vi "Write2VISA.vi"(8 "error in (no error)":errorcluster, 10 "Message_command In":T1, 11 "Command Queue In":T2) -> (0 "error out":errorcluster, 2 "Message_command Out":T1, 3 "Command Queue out":T2)   [LabVIEW 2020]
uses:
  Command_Queue.ctl
  Command_Message.ctl
  <vilib>/regexp/Match Regular Expression.xnode
panel:
  out "concatenated string":string
  out "Command":string
  out "VISA instruments":refnum<visa-resource-name>
  in  "VISA instruments":string[](array[string])=["gpib", "asrl", "com", "end of list"]
  # "end of list should be the last item"
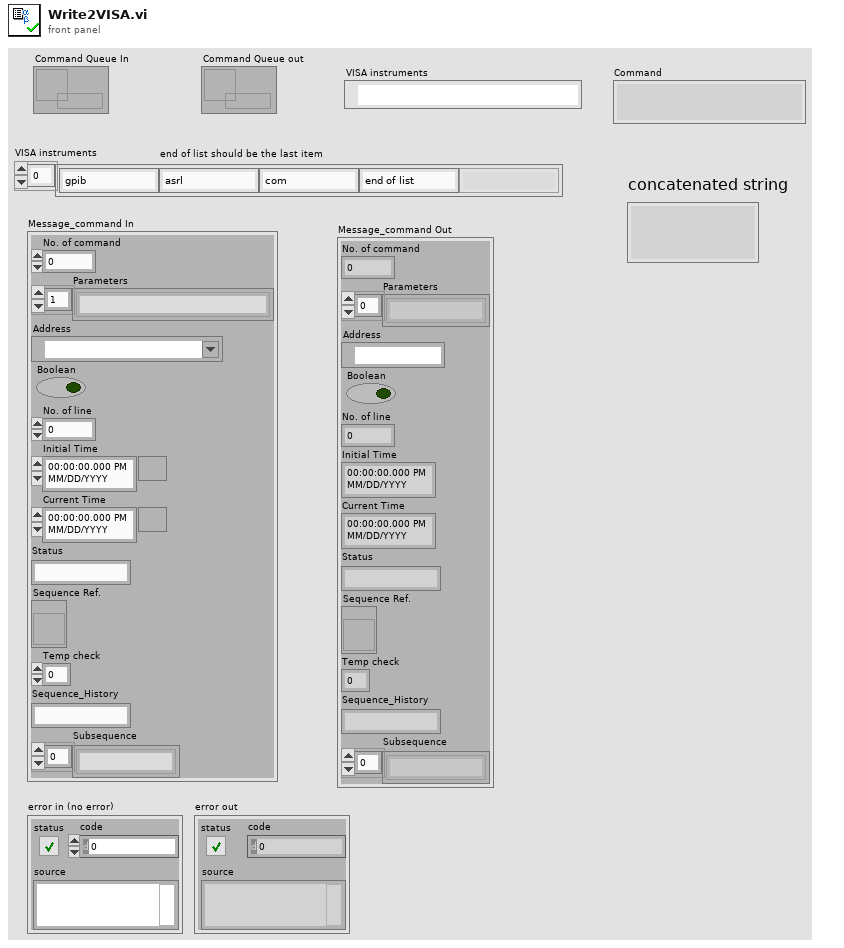
[diagram p1: front panel]
types:
  T1 = typedef "Command_Message.ctl" = cluster{"No. of command":i32, "Parameters":string[], "Address":refnum<visa-resource-name>, "Boolean":bool, "No. of line":i32, "Initial Time":timestamp, "Current Time":timestamp, "Status":string, "Sequence Ref.":refnum<vi>, "Temp check":i32, "Sequence_History":string, "Subsequence":string[]}
  T2 = typedef "Command_Queue.ctl" = refnum<queue>
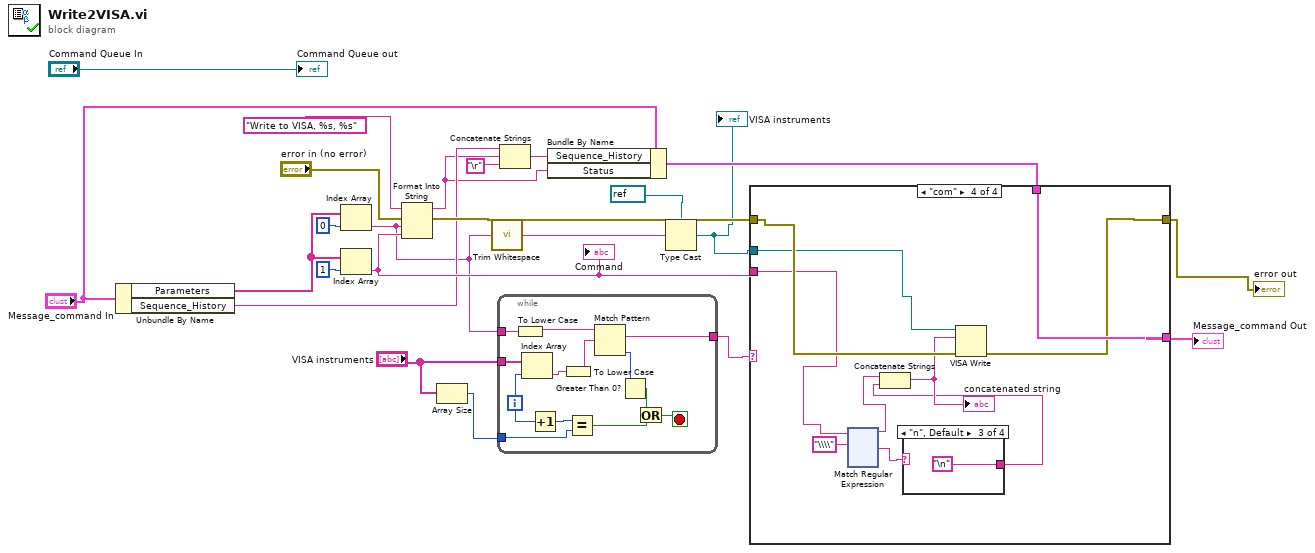
[diagram p0: block diagram]
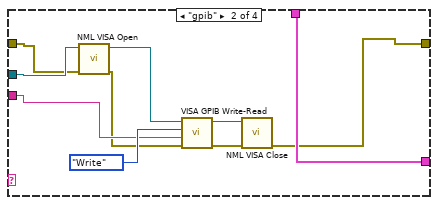
[diagram p3: hidden frame]
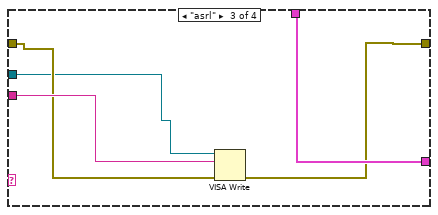
[diagram p4: hidden frame]
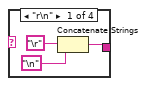
[diagram p5: hidden frame]
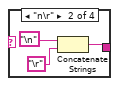
[diagram p6: hidden frame]
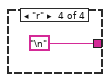
[diagram p7: hidden frame]
diagram:
  n1 = Unbundle By Name("Message_command In") -> ("Parameters"=w21:string[], "Sequence_History"=w15:string)
  n2 = Index Array(array=w21, index=0) -> (element=w5:string)
  n3 = Index Array(array=w21, index=1) -> (element=w18:string)
  "Command" <- w18
  n4 = Format Into String(format string="Write to VISA, %s, %s", error in="error in (no error)", w5, w18) -> (resulting string=w12:string, error out=w17:errorcluster)  [unwired: 1 in]
  n5 = Array Size(array="VISA instruments") -> (size(s)=w6:i32)
  n6 = call <vilib>:"Trim Whitespace.vi"("string"=w5) -> ("trimmed string"=w2:string)  [unwired: 1 in]
  n7 = while {
    tunnel: w5 -> [w36]
    tunnel: "VISA instruments" -> [w35]
    tunnel: [w30] -> w3
    tunnel: w6 -> [w25]
    i -> [w27]
    stop <- w28 stop-if-true
    n8 = To Lower Case(string=w36) -> (all lower case string=w32:string)
    n9 = Index Array(array=w35, index=w27) -> (element=w34:string)
    n10 = Increment(x=w27) -> (x+1=w26:i32)
    n11 = To Lower Case(string=w34) -> (all lower case string=w33:string)
    n12 = Equal?(x=w26, y=w25) -> (x = y?=w24:bool)
    n13 = Match Pattern(string=w32, regular expression=w33) -> (match substring=w30:string, offset past match=w31:i32)  [unwired: 1 in, 2 out]
    n14 = Greater Than 0?(x=w31) -> (x > 0?=w29:bool)
    n15 = Or(x=w29, y=w24) -> (x .or. y?=w28:bool)
  }
  n16 = Concatenate Strings(w15, w12, "\r") -> (w13:string)
  n17 = Bundle By Name(cluster="Message_command In", "Sequence_History"=w13, "Status"=w12) -> (w11:T1)
  n18 = Type Cast(type=refnum<visa-resource-name> refnum ("VISA resource name"), x=w2) -> (*(type *) &x=w1:refnum<visa-resource-name>)
  "VISA instruments" <- w1
  n19 = case shown="\"com\"" w3 {
    tunnel: w18 -> [_ w46 w52 w58]
    tunnel: w17 -> [w37 w43 w51 w62]
    tunnel: [w37 w39 w50 w61] -> w8
    tunnel: [w38 w48 w53 w63] -> w10
    tunnel: w11 -> [w38 w48 w53 w63]
    tunnel: w1 -> [_ w45 w49 w60]
    frame "end of list", Default {
    }
    frame "gpib" {
      n20 = call "NML VISA Open.vi"("error in (no error)"=w43, "VISA resource name"=w45) -> ("error out"=w42:errorcluster, "VISA resource name out"=w44:refnum<visa-resource-name>)  [unwired: 8 in]
      n21 = call "VISA GPIB Write-Read.vi"("error in (no error)"=w42, "Command"=w46, "Action"=enum16{"Write", "Read", "Write & Read"}."Write", "VISA resource name"=w44) -> ("error out"=w40:errorcluster, "dup VISA Session"=w41:refnum<visa-resource-name>)  [unwired: 4 in, 2 out]
      n22 = call "NML VISA Close.vi"("Error In"=w40, "VISA resource name"=w41) -> ("Error Out"=w39:errorcluster)  [unwired: 9 in]
    }
    frame "asrl" {
      n23 = VISA Write(VISA resource name=w49, write buffer=w52, error in (no error)=w51) -> (error out=w50:errorcluster)  [unwired: 2 out]
    }
    frame "com" {
      n24 = xnode "Match Regular Expression"("input string"=w58, "regular expression"="\\\\") -> ("before match"=w55:string, "after match"=w56:string)  [unwired: 4 in, 3 out]
      n25 = case shown="\"n\", Default" w56 {
        tunnel: [w64 w69 "\n" "\n"] -> w54
        frame "r\n" {
          n26 = Concatenate Strings("\r", "\n") -> (w64:string)
        }
        frame "n\r" {
          n27 = Concatenate Strings("\n", "\r") -> (w69:string)
        }
        frame "n", Default {
        }
        frame "r" {
        }
      }
      n28 = Concatenate Strings(w55, w54) -> (w59:string)
      "concatenated string" <- w59
      n29 = VISA Write(VISA resource name=w60, write buffer=w59, error in (no error)=w62) -> (error out=w61:errorcluster)  [unwired: 2 out]
    }
  }
  "Message_command Out" <- w10
  "error out" <- w8
  "Command Queue out" <- "Command Queue In"
